vi "Read Holding Registers.vi"(8 "error in (no error)":errorcluster, 9 "number of holding registers":u16, 10 "starting address":u16, 11 "Modbus master in":refnum<class "Modbus Master.lvclass">) -> (0 "error out":errorcluster, 2 "register values":u16[](array[numeric]), 3 "Modbus master out":refnum<class "Modbus Master.lvclass">)   [LabVIEW 2021, in "Modbus Master.lvclass"]
doc: "Reads values from contiguous holding registers. The maximum number of holding registers this VI can read is 125."
uses:
  Modbus Master.lvclass
  D:/my_projects/projects/Algorithms/Labview/21/Modbus_v1/API/Modbus API.lvclass
  Modbus Master.lvclass/Modbus Master.ctl
  Modbus API.lvclass/Modbus API.ctl
  Network Protocol/Network Master/Network Master.lvclass
  D:/my_projects/projects/Algorithms/Labview/21/Modbus_v1/Network Protocol/Network Protocol.lvclass
  Transmission Data Unit/Transmission Data Unit.lvclass
  Modbus API.lvclass
  Master Function Definition/Master Function Definition.lvclass
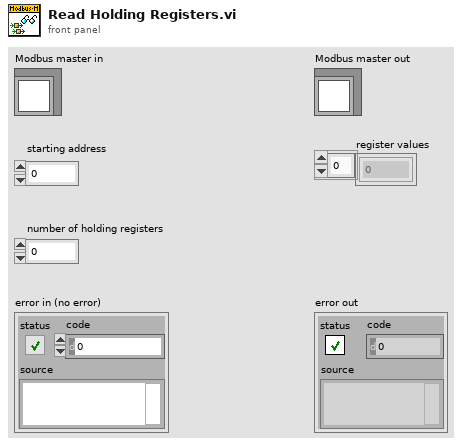
[diagram p1: front panel]
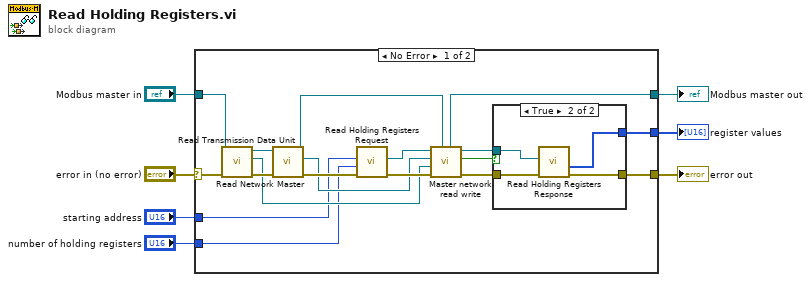
[diagram p0: block diagram]
diagram:
  n1 = case shown="No Error" "error in (no error)" {
    selector: "error in (no error)" -> [w8 w31]
    tunnel: "number of holding registers" -> [w14 _]
    tunnel: "starting address" -> [w15 _]
    tunnel: "Modbus master in" -> [w9 w32]
    tunnel: [w19 w32] -> w3
    tunnel: [w20 w31] -> w2
    tunnel: [w13 _] -> w1
    frame No Error {
      n2 = call "Read Transmission Data Unit.vi"("error in"=w8, "Modbus instance in"=w9) -> ("error out"=w25:errorcluster, "transmission data unit"=w16:refnum<class "Transmission Data Unit.lvclass">, "Modbus instance out"=w24:refnum<class "Modbus Master.lvclass">)  [unwired: 7 in]
      n3 = call "Read Network Master.vi"("error in (no error)"=w25, "Modbus master in"=w24) -> ("error out"=w21:errorcluster, "network master"=w17:refnum<class "Network Master.lvclass">, "Modbus master out"=w18:refnum<class "Modbus Master.lvclass">)  [unwired: 7 in]
      n4 = call "Read Holding Registers Request.vi"("error in"=w21, "Number of Registers"=w14, "Starting Address"=w15) -> ("error out"=w22:errorcluster, "modbus data unit out"=w11:refnum<class "Modbus Data Unit.lvclass">)  [unwired: 7 in]
      n5 = call "Master network read write.vi"("Modbus master in"=w18, "error in (no error)"=w22, "transmission data unit in"=w16, "network master in"=w17, "Modbus data unit in"=w11) -> ("error out"=w23:errorcluster, "PDU valid?"=w10:bool, "Modbus data unit out"=w12:refnum<class "Modbus Data Unit.lvclass">, "Modbus master out"=w19:refnum<class "Modbus Master.lvclass">)  [unwired: 3 in]
      n6 = case shown="True" w10 {
        tunnel: w23 -> [w26 w30]
        tunnel: [w26 w29] -> w20
        tunnel: [_ w28] -> w13
        tunnel: w12 -> [_ w27]
        frame False {
        }
        frame True {
          n7 = call "Read Holding Registers Response.vi"("error in"=w30, "modbus data unit in"=w27) -> ("error out"=w29:errorcluster, "Register Values"=w28:u16[])  [unwired: 7 in, 1 out]
        }
      }
    }
    frame Error {
    }
  }
  "Modbus master out" <- w3
  "error out" <- w2
  "register values" <- w1
